vi "Main.vi"() -> ()   [LabVIEW 2019]
uses:
  Global.vi
  <vilib>/Utility/file.llb/Read Delimited Spreadsheet (DBL).vi
panel:
  out "Absorbancs Graph":cluster{dbl[], dbl[]}[](graph)=[{[210.47, 211.013, 211.556, 212.099, 212.642, 213.185, 213.728, 214.271, 214.814, 215.357, 215.9, 216.443, 216.986, 217.529, 218.072, 218.615, 219.158, 219.701, 220.244, 220.787, 221.33, 221.873, 222.416, 222.959, 223.502, 224.045, 224.588, 225.131, 225.674, 226.217, 226.76, 227.303, 227.846, 228.389, 228.932, 229.475, 230.018, 230.561, 231.104, 231.647, 232.19, 232.733, 233.276, 233.819, 234.362, 234.905, 235.448, 235.991, 236.534, 237.077, 237.62, 238.163, 238.706, 239.249, 239.792, 240.335, 240.878, 241.421, 241.964, 242.507, 243.05, 243.593, 244.136, 244.679, 245.222, 245.765, 246.308, 246.851, 247.394, 247.937, 248.48, 249.023, 249.566, 250.109, 250.652, 251.195, 251.738, 252.281, 252.824, 253.367, 253.91, 254.453, 254.996, 255.539, 256.082, 256.625, 257.168, 257.711, 258.254, 258.797, 259.34, 259.883], [0.859775678286318, 0.8194318156296146, 0.7895662441158913, 0.7653583418970374, 0.7134020372603199, 0.6674930001591154, 0.6169042198464642, 0.5666594591614739, 0.5127610913357338, 0.4760432747417854, 0.43179210618385533, 0.39546521483677954, 0.35704563080021307, 0.3204937163802063, 0.2943543872023645, 0.2644968000756883, 0.23727151168709026, 0.21506292164762564, 0.19582373256481655, 0.17509578429484746, 0.15778012766612576, 0.14182714481381176, 0.12762613288942176, 0.11359011007339652, 0.10311798710231297, 0.0919810390323458, 0.08407740857125809, 0.07520310011257239, 0.06894533118889845, 0.06156116409513224, 0.054721465538073055, 0.04951119044573565, 0.04379079748078188, 0.040522877073344524, 0.03583986731239025, 0.03120271181313547, 0.02776368982361145, 0.024890944782316078, 0.021970298789674186, 0.019046917639680402, 0.017650784209329966, 0.014430138184920574, 0.012660635378348474, 0.010678518980179588, 0.00996203492854495, 0.00865803175790969, 0.007123137178893124, 0.006459897966245347, 0.005454774486390257, 0.004673433507016052, 0.00317899640396703, 0.002978638971630067, 0.0032063812554244536, 0.0025374593715086283, 0.0010371917010740805, 0.0013682683081331706, 0.0012338025827769855, 0.00044231588608750066, 0.0006576235447054053, 0.0003592638366740966, 3.86590865093725e-05, -5.462381588621987e-05, -0.00043697341233217557, 0.00028768565388054973, -0.0005029989692543549, -0.0003836845555745434, -2.1769830005107654e-05, -8.158566931395356e-05, -0.0012657429248070888, -0.0009881653780830016, -0.0006206450872670022, -0.0008460195763415369, -0.0008440728182035687, -0.0008541442548795249, 0.0003212150192799558, -0.00016824964081266214, -0.0006849404823446592, 0.0004342318774892516, 0.00025692780195036777, 0.00010544427557851802, 0.00044687325757008026, -0.00017318641138520594, -4.097812470797019e-05, -8.4835930852626e-05, -0.00032452033611190395, -0.0006147450240710922, 0.00011997159689319109, -0.00015409533396294056, 0.0006683040427777585, 0.00014999181500151976, 0.0010128166761367956, 0.0012425823150642307]}, {[210.47, 211.013, 211.556, 212.099, 212.642, 213.185, 213.728, 214.271, 214.814, 215.357, 215.9, 216.443, 216.986, 217.529, 218.072, 218.615, 219.158, 219.701, 220.244, 220.787, 221.33, 221.873, 222.416, 222.959, 223.502, 224.045, 224.588, 225.131, 225.674, 226.217, 226.76, 227.303, 227.846, 228.389, 228.932, 229.475, 230.018, 230.561, 231.104, 231.647, 232.19, 232.733, 233.276, 233.819, 234.362, 234.905, 235.448, 235.991, 236.534, 237.077, 237.62, 238.163, 238.706, 239.249, 239.792, 240.335, 240.878, 241.421, 241.964, 242.507, 243.05, 243.593, 244.136, 244.679, 245.222, 245.765, 246.308, 246.851, 247.394, 247.937, 248.48, 249.023, 249.566, 250.109, 250.652, 251.195, 251.738, 252.281, 252.824, 253.367, 253.91, 254.453, 254.996, 255.539, 256.082, 256.625, 257.168, 257.711, 258.254, 258.797, 259.34, 259.883], [0.801341170479744, 0.7542734132237421, 0.6980568093186122, 0.65420605249337, 0.591680060881281, 0.5299625392926228, 0.47702592078260647, 0.4255234062398998, 0.3711647669162868, 0.3228829251218208, 0.2827599748503002, 0.2434409059716668, 0.2119311833930049, 0.1798378791449536, 0.15402672866461736, 0.13094215234558915, 0.10931855345881111, 0.09491646684250218, 0.07742521143320874, 0.06462685612767415, 0.05592972771866379, 0.04553833460727783, 0.03699743050859016, 0.031488515184952236, 0.025748999955385175, 0.020904706258801094, 0.018642890097352365, 0.013432623513669001, 0.010553223074843139, 0.009115474310373156, 0.008106302412446732, 0.00717074031072442, 0.005744777726777169, 0.004893684096016718, 0.0031711878437890757, 0.0015769760381964641, 0.0017569164268725172, 0.001484919073282149, 0.00034167784506089136, 0.00042709614687959363, -0.00019894237181035043, -0.0002881289314805198, -0.0009673652556734837, -0.0011091138604324736, 0.000146281936226407, -0.0005078123746470216, -0.0006453921276296619, -0.00040921704838469547, -0.00025853371894282023, -5.8841081421987657e-05, -0.0008455489737523095, -0.0003666006559215444, -0.0001741794938470015, -9.572694367300863e-05, -0.00013418443402012092, -0.0004342119920670712, -2.785591609676813e-05, -0.0005634379748792259, 0.0004540623443782983, -5.8901234707184336e-05, -0.00013105680029032452, -0.0003600499082511144, -0.0003055170322483515, 0.00045608059860526365, -0.00013473988615758312, 0.0007354698007963102, 0.00032433285193672265, 0.0007906108278793178, 7.605421447198432e-05, 8.534654960939622e-05, 0.0006625762183634851, -0.0005709729804337961, -0.0010150816524892026, 0.0001368035849654524, -0.000687954722901625, -0.00014905489719789847, 0.00011942950940802693, 0.000443837174362572, 0.00026005063494623573, -0.00020446941719183195, 0.000928426415228837, 0.000149226286241394, 2.9499413362117644e-05, -4.747285768441287e-05, 0.00033451056635025456, -0.00033948938772015297, -0.00025802686603175473, -0.0010796627525889724, 8.508559467040183e-05, 0.00019199329640829516, -2.422754560728671e-05, 0.00012878794244869374]}, {[210.47, 211.013, 211.556, 212.099, 212.642, 213.185, 213.728, 214.271, 214.814, 215.357, 215.9, 216.443, 216.986, 217.529, 218.072, 218.615, 219.158, 219.701, 220.244, 220.787, 221.33, 221.873, 222.416, 222.959, 223.502, 224.045, 224.588, 225.131, 225.674, 226.217, 226.76, 227.303, 227.846, 228.389, 228.932, 229.475, 230.018, 230.561, 231.104, 231.647, 232.19, 232.733, 233.276, 233.819, 234.362, 234.905, 235.448, 235.991, 236.534, 237.077, 237.62, 238.163, 238.706, 239.249, 239.792, 240.335, 240.878, 241.421, 241.964, 242.507, 243.05, 243.593, 244.136, 244.679, 245.222, 245.765, 246.308, 246.851, 247.394, 247.937, 248.48, 249.023, 249.566, 250.109, 250.652, 251.195, 251.738, 252.281, 252.824, 253.367, 253.91, 254.453, 254.996, 255.539, 256.082, 256.625, 257.168, 257.711, 258.254, 258.797, 259.34, 259.883], [0.8349250299196103, 0.7985659782220785, 0.7554294716845671, 0.7039073271955195, 0.6643155846589284, 0.6159979981150474, 0.5705818180332749, 0.5241666942013795, 0.4664351446159479, 0.4314871898047554, 0.3889092668584453, 0.35397500896861966, 0.32082659223672977, 0.29058708622423546, 0.26100520078520395, 0.23636505571931815, 0.212374355658777, 0.1941007847601965, 0.17582536275176977, 0.15957915032302233, 0.14560551256364115, 0.13224949336973374, 0.11922368957919263, 0.1097629242038428, 0.10189705539077057, 0.0928971760093605, 0.08538635126587726, 0.07812652408738596, 0.07171836378664848, 0.06508217851129808, 0.060563676829728776, 0.0558150422512567, 0.052404168918151785, 0.04734459073599655, 0.043400995888894185, 0.03996295459186795, 0.03540756730509166, 0.033186749038576574, 0.029867698307559296, 0.027606079350583596, 0.024793568873241023, 0.02179476713041542, 0.019525144001637858, 0.01779689632707871, 0.016386094716066633, 0.014686993002350365, 0.012953061761290088, 0.011800535044244484, 0.009986607793191861, 0.008508683009597853, 0.007255921855678818, 0.005920522311633751, 0.005428452139574033, 0.004341510976025073, 0.003272882804573607, 0.002792275615607423, 0.002627046818162858, 0.001956247104735409, 0.001975511612610885, 0.0005299670100274712, 0.0004937405679766166, 0.0010159557259308144, -0.00043008610603853525, 0.00022898969989317702, -0.0009699640550975969, 5.282040887574779e-05, -0.0010025972441931735, -0.0006509174041809049, -0.0017295119228779299, -0.0026943110513844987, -0.0017292772649578902, -0.0011740793412730113, -0.0020890149910946926, -0.0026277233640298464, -0.0007945791770674893, -0.0006339544985643902, -0.0012460337713899386, -0.0006416045454584116, -0.0004387120217184681, -0.0007055787813360359, -0.00044316594100983486, -0.0006635248767982091, -0.0009792362292916634, -0.00013667933511483932, 0.0006261275336703967, -0.0005395860806047259, 0.00012159334130024124, 0.0010251084460011217, 0.0018025827427642638, 0.001831767211735412, 0.0024732113092995472, 0.002767192854815498]}]
  out "A'- Graph":cluster{dbl[], dbl[]}[](graph)=[{[210.47, 211.013, 211.556, 212.099, 212.642, 213.185, 213.728, 214.271, 214.814, 215.357, 215.9, 216.443, 216.986, 217.529, 218.072, 218.615, 219.158, 219.701, 220.244, 220.787, 221.33, 221.873, 222.416, 222.959, 223.502, 224.045, 224.588, 225.131, 225.674, 226.217, 226.76, 227.303, 227.846, 228.389, 228.932, 229.475, 230.018, 230.561, 231.104, 231.647, 232.19, 232.733, 233.276, 233.819, 234.362, 234.905, 235.448, 235.991, 236.534, 237.077, 237.62, 238.163, 238.706, 239.249, 239.792, 240.335, 240.878, 241.421, 241.964, 242.507, 243.05, 243.593, 244.136, 244.679, 245.222, 245.765, 246.308, 246.851, 247.394, 247.937, 248.48, 249.023, 249.566, 250.109, 250.652, 251.195, 251.738, 252.281, 252.824, 253.367, 253.91, 254.453, 254.996, 255.539, 256.082, 256.625, 257.168, 257.711, 258.254, 258.797, 259.34, 259.883], [0.12793016694096082, 0.1327881561828641, 0.13898634561838696, 0.12591972077414348, 0.14132650024267335, 0.14734372113403094, 0.1485442487837778, 0.14751986962096558, 0.1377505703158608, 0.1454257108067617, 0.13827874574091015, 0.1380955602332684, 0.13280214091499964, 0.13096155295962345, 0.1242263335792905, 0.12003173950478929, 0.11520703411258498, 0.10969549971555984, 0.1069423396107689, 0.10205574991791058, 0.09580016806982122, 0.09167882996708734, 0.08624690930416284, 0.08168334522252357, 0.07892496597610259, 0.07423828091165904, 0.06873855259983945, 0.06612583621347973, 0.06228574814736767, 0.056930857187937944, 0.05331141850375127, 0.049396798883806, 0.04725985884383318, 0.042960378591267154, 0.040558634335614574, 0.038548841416862094, 0.03383136521287019, 0.031853948056984105, 0.02956088014857819, 0.027222379512650333, 0.02497238017948171, 0.02205386048567311, 0.02039542923280995, 0.01879516854143684, 0.016254370606103935, 0.015144480862862991, 0.013534765266055699, 0.012169541069378806, 0.01021984544175458, 0.008561791484343755, 0.008019447576661586, 0.006251714332178242, 0.0055858813703053, 0.004428072374523385, 0.0033942758849625923, 0.0031852781299558422, 0.0026522707441254765, 0.0024666851934537033, 0.001563969608097927, 0.0005833772835681486, 0.0006126350464351532, 0.0013427440658959052, -0.0001526640434080166, -0.00018534269449400133, -0.0008475009717322837, -0.0006159477395225684, -0.0012976525297084872, -0.0013704938482608704, -0.001798765017845805, -0.0027720616232884314, -0.0023331635827748016, -0.0006534404274150182, -0.0011629877379098984, -0.0027525829787817795, -0.00016639630496898027, -0.0004977867659968762, -0.0013551881915035838, -0.0010474447563982889, -0.000676610158729499, -0.0005184402556335553, -0.0012932934214892246, -0.000800229631418983, -0.001006272911124815, -9.314949136806912e-05, 0.0003192583376444662, -0.00022800478420321665, 0.00035851885260999834, 0.00201693730327079, 0.0017243828096380077, 0.001655229240884793, 0.002495498904283519, 0.002648662191671046]}]
  out "ENo3- Graph":cluster{dbl[], dbl[]}[](graph)=[{[210.47, 211.013, 211.556, 212.099, 212.642, 213.185, 213.728, 214.271, 214.814, 215.357, 215.9, 216.443, 216.986, 217.529, 218.072, 218.615, 219.158, 219.701, 220.244, 220.787, 221.33, 221.873, 222.416, 222.959, 223.502, 224.045, 224.588, 225.131, 225.674, 226.217, 226.76, 227.303, 227.846, 228.389, 228.932, 229.475, 230.018, 230.561, 231.104, 231.647, 232.19, 232.733, 233.276, 233.819, 234.362, 234.905, 235.448, 235.991, 236.534, 237.077, 237.62, 238.163, 238.706, 239.249, 239.792, 240.335, 240.878, 241.421, 241.964, 242.507, 243.05, 243.593, 244.136, 244.679, 245.222, 245.765, 246.308, 246.851, 247.394, 247.937, 248.48, 249.023, 249.566, 250.109, 250.652, 251.195, 251.738, 252.281, 252.824, 253.367, 253.91, 254.453, 254.996, 255.539, 256.082, 256.625, 257.168, 257.711, 258.254, 258.797, 259.34, 259.883], [2945.330127801271, 2980.855275880313, 3436.2790959666113, 3769.744784933901, 3866.894510497265, 4084.8736146849583, 4023.379959193408, 3942.792626230383, 3841.4870174255007, 4000.655053294645, 3828.2175896632853, 3817.29963026311, 3602.043449269673, 3441.6817617479314, 3385.4779019137154, 3191.9094774780338, 3027.900988481217, 2827.916240006436, 2758.161391723025, 2559.4402139484487, 2352.543562902859, 2211.319435258279, 2071.254044684568, 1872.4985984661555, 1757.9755053965123, 1610.3756628618062, 1481.2220799419745, 1391.9041799350034, 1312.4602246379604, 1178.0792525407564, 1046.9242425921682, 950.4885917176833, 853.0143961733057, 798.0735127864109, 729.9870960192372, 660.3096910237371, 580.0703495049484, 521.9091337484808, 481.03639003988167, 414.2641235694944, 396.4369339279932, 326.7555408020507, 301.8030154403679, 260.7798205817484, 218.2783416579434, 203.17512601786376, 172.00088731688328, 152.2553896286287, 126.72119927733758, 105.10817416921849, 88.68612370915851, 74.02308578565034, 74.9778366321423, 58.43746750873835, 25.92479027667191, 39.72329096416452, 28.016242550079305, 21.946810990329947, 4.837550849460239, 9.253260306661115, 3.6872160631477606, 6.564562628975335, -3.102759697380701, -3.4822870243873694, -8.257001809816265, -24.48707752878695, -7.530208161604536, -19.009160404506808, -29.78370140188913, -23.819749647347457, -28.252299308214194, -6.325350510303438, 3.4461920657718994, -21.976730977680553, 22.220061147224676, -0.46747996303027756, -17.84505210776972, -0.11357589657642167, -0.01733438945422087, 6.851118545455417, -10.561490174616834, -7.145991484163017, -1.5631996144296523, -0.8338814015497948, -14.628189953991297, -6.125489805889719, 8.399819289346626, 20.594630435447556, 12.956187847181663, -0.9477195505370489, 23.047848091745728, 24.73487218805406]}]
  out "[NO3] Linear fit":dbl=39.51302180661577 format="%#_3g"
  in  "Path Length":dbl=1.0 format="%#_13g"
  in  "[NO3-]":dbl=4.5e-05 caption="Known Nitrate Concentration"
  in  "S(TS)":dbl=33.66 caption="Sample Water Salinity" format="%#_13g"
  in  "S(KN)":dbl=33.85 caption="Calibration Salinity" format="%#_13g"
  in  "T(KN)":dbl=21.0 caption="Calibration Temp Zero Nitrate" format="%#_13g"
  in  "S(Norm)":dbl=35.0 caption="Calibration Salinity" format="%#_13g"
  in  "T(TS)":dbl=20.0 caption="Test Sample Sea Water Temp" format="%#_13g"
  in  "T(ZN)":dbl=19.3 caption="Calibration Temp Zero Nitrate" format="%#_13g"
  in  "S(ZN)":dbl=36.052 caption="Zero Nitrate Sea Water  Salinity" format="%#_13g"
  in  "btnCalcNitrate":bool caption="Calculate Nitrate"
  in  "DAC":T1(tab)
  in  "numTS":i32=6 caption="Column # (Zero Indexed)"
  in  "numKN":i32=3 caption="Column # (Zero Indexed)"
  in  "numZN":i32=4 caption="Column # (Zero Indexed)"
  in  "numDI":i32=2 caption="Column # (Zero Indexed)"
  in  "numDark":i32=1 caption="Column # (Zero Indexed)"
  out "ledTS":bool caption="Done"
  out "ledKN":bool caption="Done"
  out "ledZN":bool caption="Done"
  out "ledDI":bool caption="Done"
  out "ledDark":bool caption="Done"
  in  "Path":path=path "C:/Users/Omid/Desktop/SIO 179/Nitrate/SIO179NitrateCalc/Data/DataSampled(11-12).csv"
  in  "btnReadFromFile":bool caption="Read from CSV file"
  out "Intensity Signal Graph":cluster{dbl[], dbl[]}[](graph)
  out "Intensity Graph":cluster{dbl[], dbl[]}[](graph)=[{[210.47, 211.013, 211.556, 212.099, 212.642, 213.185, 213.728, 214.271, 214.814, 215.357, 215.9, 216.443, 216.986, 217.529, 218.072, 218.615, 219.158, 219.701, 220.244, 220.787, 221.33, 221.873, 222.416, 222.959, 223.502, 224.045, 224.588, 225.131, 225.674, 226.217, 226.76, 227.303, 227.846, 228.389, 228.932, 229.475, 230.018, 230.561, 231.104, 231.647, 232.19, 232.733, 233.276, 233.819, 234.362, 234.905, 235.448, 235.991, 236.534, 237.077, 237.62, 238.163, 238.706, 239.249, 239.792, 240.335, 240.878, 241.421, 241.964, 242.507, 243.05, 243.593, 244.136, 244.679, 245.222, 245.765, 246.308, 246.851, 247.394, 247.937, 248.48, 249.023, 249.566, 250.109, 250.652, 251.195, 251.738, 252.281, 252.824, 253.367, 253.91, 254.453, 254.996, 255.539, 256.082, 256.625, 257.168, 257.711, 258.254, 258.797, 259.34, 259.883], [2945.330127801271, 2980.855275880313, 3436.2790959666113, 3769.744784933901, 3866.894510497265, 4084.8736146849583, 4023.379959193408, 3942.792626230383, 3841.4870174255007, 4000.655053294645, 3828.2175896632853, 3817.29963026311, 3602.043449269673, 3441.6817617479314, 3385.4779019137154, 3191.9094774780338, 3027.900988481217, 2827.916240006436, 2758.161391723025, 2559.4402139484487, 2352.543562902859, 2211.319435258279, 2071.254044684568, 1872.4985984661555, 1757.9755053965123, 1610.3756628618062, 1481.2220799419745, 1391.9041799350034, 1312.4602246379604, 1178.0792525407564, 1046.9242425921682, 950.4885917176833, 853.0143961733057, 798.0735127864109, 729.9870960192372, 660.3096910237371, 580.0703495049484, 521.9091337484808, 481.03639003988167, 414.2641235694944, 396.4369339279932, 326.7555408020507, 301.8030154403679, 260.7798205817484, 218.2783416579434, 203.17512601786376, 172.00088731688328, 152.2553896286287, 126.72119927733758, 105.10817416921849, 88.68612370915851, 74.02308578565034, 74.9778366321423, 58.43746750873835, 25.92479027667191, 39.72329096416452, 28.016242550079305, 21.946810990329947, 4.837550849460239, 9.253260306661115, 3.6872160631477606, 6.564562628975335, -3.102759697380701, -3.4822870243873694, -8.257001809816265, -24.48707752878695, -7.530208161604536, -19.009160404506808, -29.78370140188913, -23.819749647347457, -28.252299308214194, -6.325350510303438, 3.4461920657718994, -21.976730977680553, 22.220061147224676, -0.46747996303027756, -17.84505210776972, -0.11357589657642167, -0.01733438945422087, 6.851118545455417, -10.561490174616834, -7.145991484163017, -1.5631996144296523, -0.8338814015497948, -14.628189953991297, -6.125489805889719, 8.399819289346626, 20.594630435447556, 12.956187847181663, -0.9477195505370489, 23.047848091745728, 24.73487218805406]}]
  out "ledSampledStatus":bool caption="Sampling is done!!"
  in  "Variable Selector":string(combo)="Dark Signal"
  in  "btnSampleFromSpectrometer":bool caption="Sample Signal From Spectrometer"
  out "ledSalinitySampledStatus":bool caption="Sampling is done!"
  in  "cmbSalinityVariableSelector":string(combo) caption="Variable Selector"
  in  "btnReadFromSalinitySensor":bool caption="Read from Salinity sensor"
  in  "baud rate":u32=9600 caption="Baud Rate"
  in  "Port Name":refnum<visa-resource-name>="COM1"
  in  "stop":bool
  # "Dark Signal"
  # "DI Water Signal"
  # "Zero Nitrate Signal"
  # "Known Nitrate Signal"
  # "Test Sample Signal"
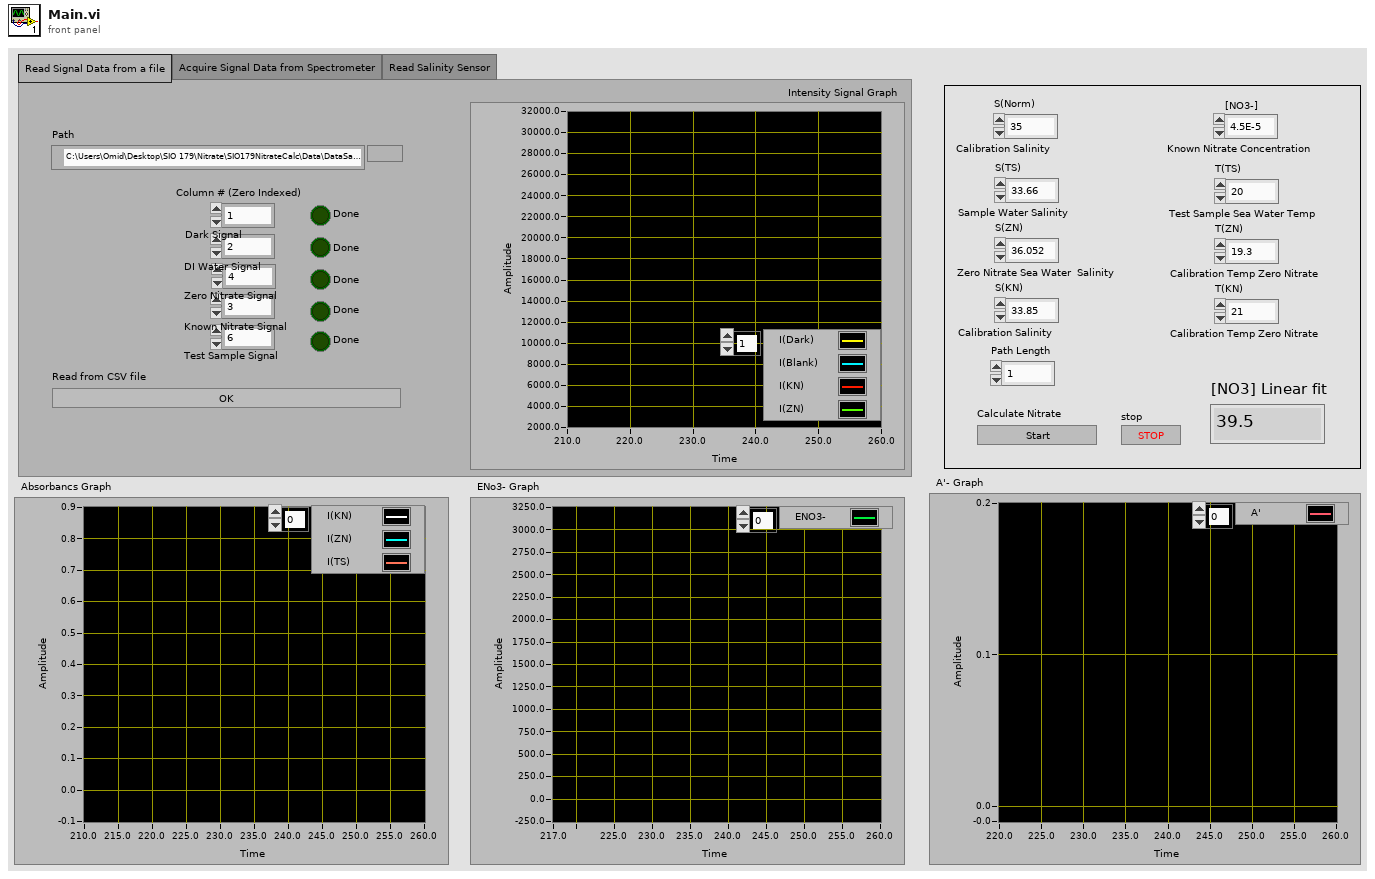
[diagram p1: front panel]
types:
  T1 = enum32{"Read Signal Data from a file", "Acquire Signal Data from Spectrometer", "Read Salinity Sensor"}
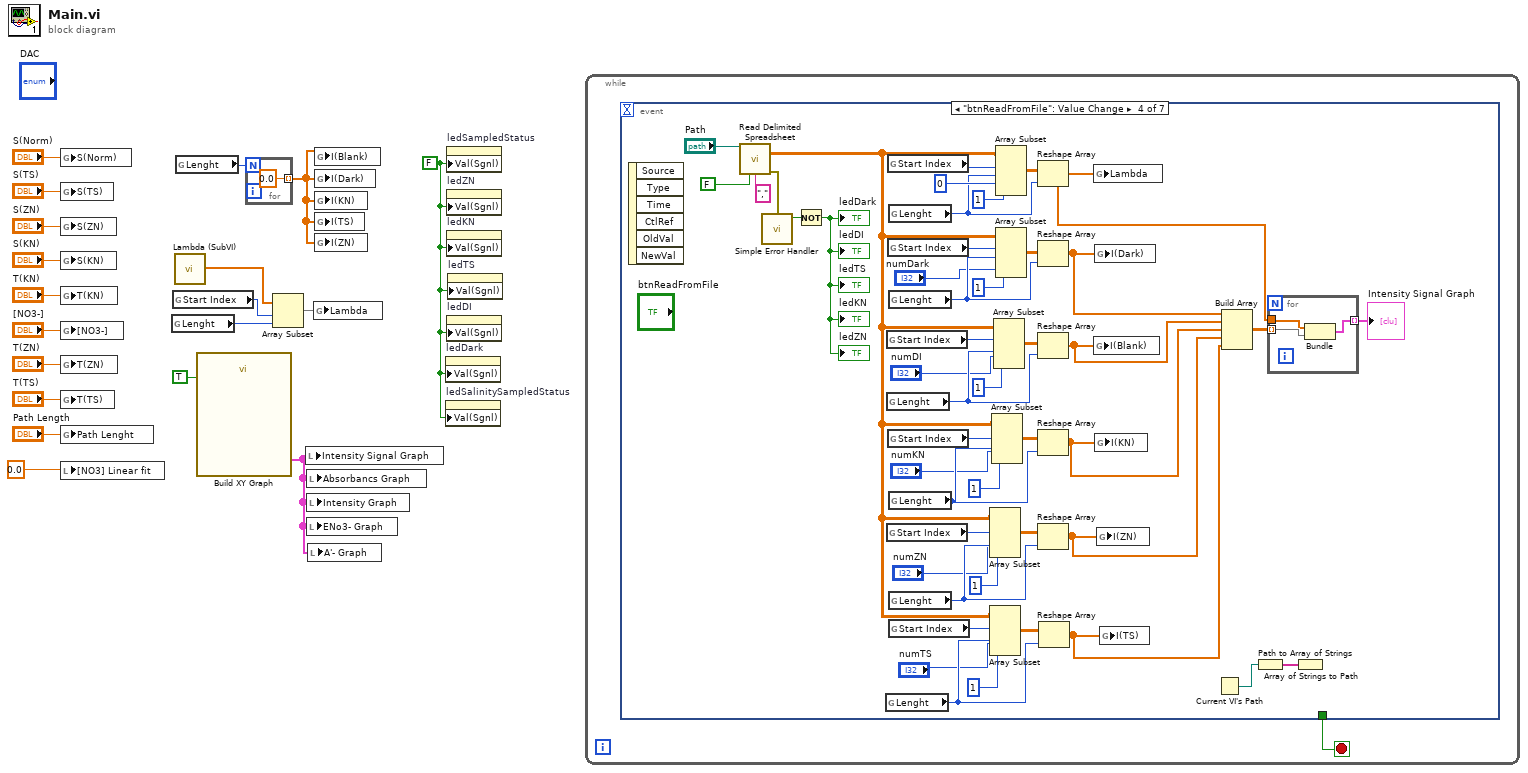
[diagram p0: block diagram]
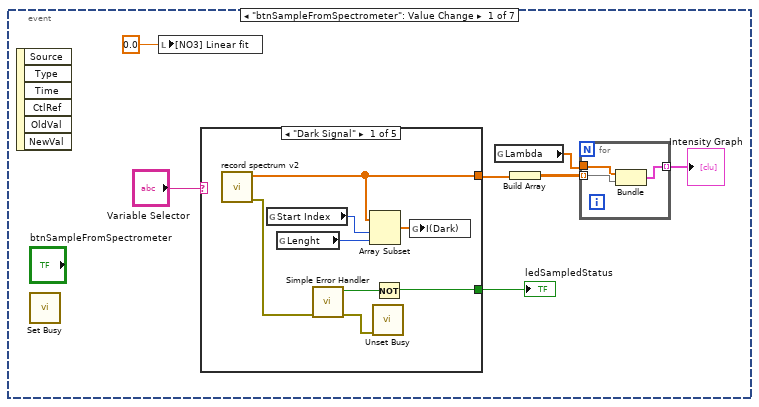
[diagram p2: hidden frame]
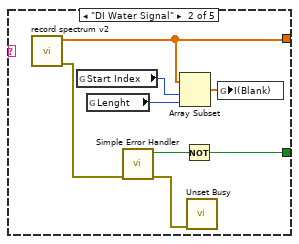
[diagram p3: hidden frame]
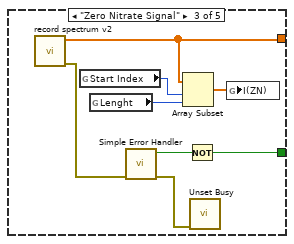
[diagram p4: hidden frame]
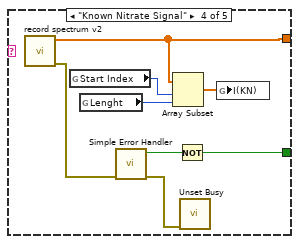
[diagram p5: hidden frame]
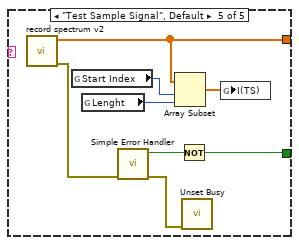
[diagram p6: hidden frame]
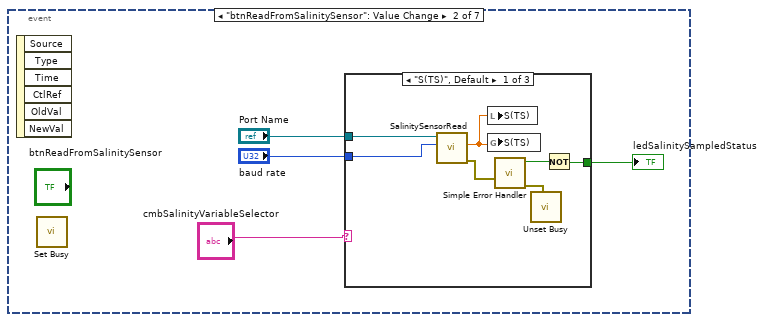
[diagram p7: hidden frame]
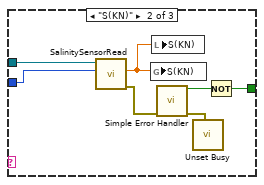
[diagram p8: hidden frame]
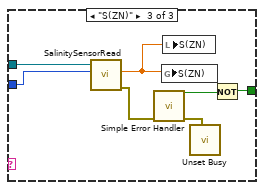
[diagram p9: hidden frame]
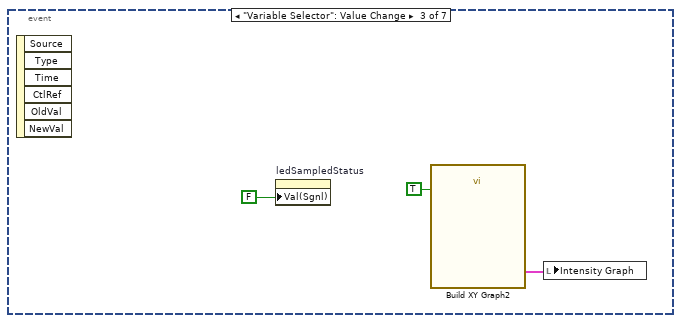
[diagram p10: hidden frame]
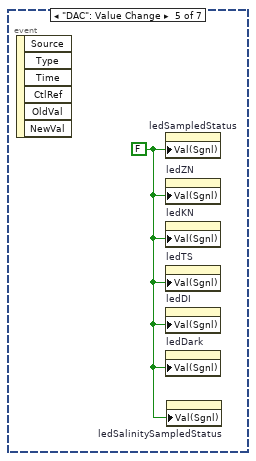
[diagram p11: hidden frame]
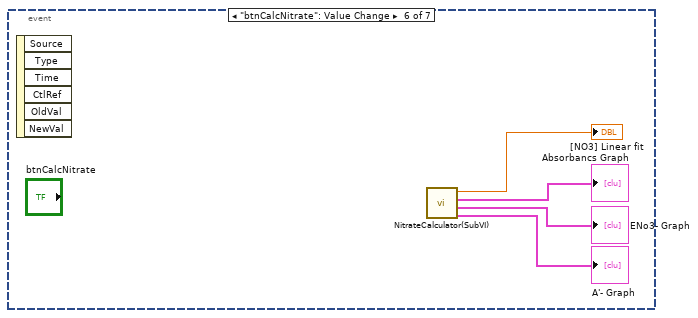
[diagram p12: hidden frame]
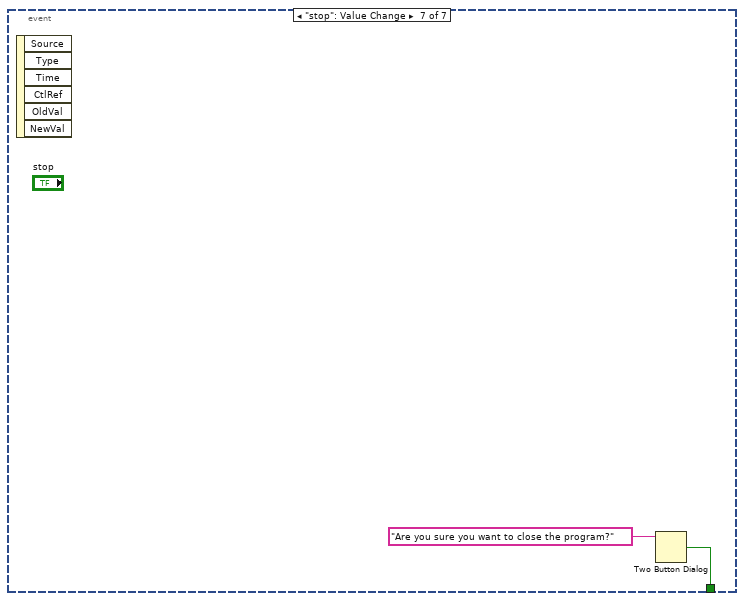
[diagram p13: hidden frame]
diagram:
  w10 = FALSE ("Value (Signaling)")
  n1 = global write "Global.vi" "S(Norm)"("S(Norm)") -> ()
  n2 = global write "Global.vi" "S(TS)"("S(TS)") -> ()
  n3 = global write "Global.vi" "S(ZN)"("S(ZN)") -> ()
  n4 = global write "Global.vi" "S(KN)"("S(KN)") -> ()
  n5 = global write "Global.vi" "T(KN)"("T(KN)") -> ()
  n6 = global write "Global.vi" "[NO3-]"("[NO3-]") -> ()
  n7 = global write "Global.vi" "T(ZN)"("T(ZN)") -> ()
  n8 = global write "Global.vi" "T(TS)"("T(TS)") -> ()
  n9 = global write "Global.vi" "Path Lenght"("Path Length") -> ()
  n10 = local write "[NO3] Linear fit"(0.0 ("[NO3] Linear fit")) -> ()
  n11 = global read "Global.vi" "Lenght"() -> (w16:i32)
  n12 = global read "Global.vi" "Start Index"() -> (w15:i32)
  n13 = call "Lambda (SubVI).vi"() -> ("Lambda"=w13:dbl[])  [unwired: 11 in]
  n14 = global read "Global.vi" "Lenght"() -> (w12:i32)
  n15 = call "Build XY Graph"("Reset"=TRUE) -> ("XY Graph"=w19:cluster{"Y":dbl[], "Y":dbl[]}[])  [unwired: 4 in, 6 out]
  n16 = for {
    N: w12 -> [_]
    tunnel: [0.0] -> w11 mode=indexing
  }
  n17 = Array Subset(array=w13, index=w15, length=w16) -> (w14:dbl[])
  n18 = local write "Intensity Signal Graph"(w19) -> ()
  n19 = local write "Absorbancs Graph"(w19) -> ()
  n20 = local write "Intensity Graph"(w19) -> ()
  n21 = local write "ENo3- Graph"(w19) -> ()
  n22 = local write "A'- Graph"(w19) -> ()
  n23 = global write "Global.vi" "Lambda"(w14) -> ()
  n24 = global write "Global.vi" "I(Blank)"(w11) -> ()
  n25 = global write "Global.vi" "I(Dark)"(w11) -> ()
  n26 = global write "Global.vi" "I(KN)"(w11) -> ()
  n27 = global write "Global.vi" "I(TS)"(w11) -> ()
  n28 = global write "Global.vi" "I(ZN)"(w11) -> ()
  n29 = property on="ledDark" class="Bool (strict)"("Val(Sgnl)"=w10) -> ()  [unwired: 2 in, 2 out]
  n30 = property on="ledSalinitySampledStatus" class="Bool (strict)"("Val(Sgnl)"=w10) -> ()  [unwired: 2 in, 2 out]
  n31 = property on="ledSampledStatus" class="Bool (strict)"("Val(Sgnl)"=w10) -> ()  [unwired: 2 in, 2 out]
  n32 = property on="ledZN" class="Bool (strict)"("Val(Sgnl)"=w10) -> ()  [unwired: 2 in, 2 out]
  n33 = property on="ledKN" class="Bool (strict)"("Val(Sgnl)"=w10) -> ()  [unwired: 2 in, 2 out]
  n34 = property on="ledDI" class="Bool (strict)"("Val(Sgnl)"=w10) -> ()  [unwired: 2 in, 2 out]
  n35 = property on="ledTS" class="Bool (strict)"("Val(Sgnl)"=w10) -> ()  [unwired: 2 in, 2 out]
  n36 = while {
    stop <- w21 stop-if-true
    n37 = event shown="[3] \"btnReadFromFile\": Value Change" {
      selector: _ -> [_ _ _ _ _ _ _]
      dyn-events: _ -> [_ _ _ _ _ _ _]
      timeout: _ -> [_ _ _ _ _ _ _]
      tunnel: [_ _ _ _ _ _ w156] -> w21
      event "btnSampleFromSpectrometer": Value Change {
        n38 = event-data() -> ()  [unwired: 1 in, 6 out]
        n39 = call <vilib>:"Set Busy.vi"() -> ()  [unwired: 10 in, 2 out]
        n40 = local write "[NO3] Linear fit"(0.0 ("[NO3] Linear fit")) -> ()
        n41 = case shown="\"Dark Signal\"" "Variable Selector" {
          tunnel: [w32 w40 w48 w56 w70] -> w27
          tunnel: [w33 w41 w49 w57 w64] -> w24
          frame "Dark Signal" {
            n42 = call "record spectrum v2.vi"() -> ("error out"=w36:errorcluster, "Array"=w33:dbl[])  [unwired: 9 in, 1 out]
            n43 = global read "Global.vi" "Start Index"() -> (w37:i32)
            n44 = global read "Global.vi" "Lenght"() -> (w38:i32)
            n45 = call <vilib>:"Simple Error Handler.vi"("error in (no error)"=w36) -> ("error?"=w34:bool, "error out"=w35:errorcluster)  [unwired: 4 in, 3 out]
            n46 = Array Subset(array=w33, index=w37, length=w38) -> (w39:dbl[])
            n47 = call <vilib>:"Unset Busy.vi"("error in (no error)"=w35) -> ()  [unwired: 10 in, 1 out]
            n48 = Not(x=w34) -> (.not. x?=w32:bool)
            n49 = global write "Global.vi" "I(Dark)"(w39) -> ()
          }
          frame "DI Water Signal" {
            n50 = call "record spectrum v2.vi"() -> ("error out"=w45:errorcluster, "Array"=w41:dbl[])  [unwired: 9 in, 1 out]
            n51 = global read "Global.vi" "Start Index"() -> (w44:i32)
            n52 = global read "Global.vi" "Lenght"() -> (w43:i32)
            n53 = call <vilib>:"Simple Error Handler.vi"("error in (no error)"=w45) -> ("error?"=w47:bool, "error out"=w46:errorcluster)  [unwired: 4 in, 3 out]
            n54 = Array Subset(array=w41, index=w44, length=w43) -> (w42:dbl[])
            n55 = Not(x=w47) -> (.not. x?=w40:bool)
            n56 = call <vilib>:"Unset Busy.vi"("error in (no error)"=w46) -> ()  [unwired: 10 in, 1 out]
            n57 = global write "Global.vi" "I(Blank)"(w42) -> ()
          }
          frame "Zero Nitrate Signal" {
            n58 = call "record spectrum v2.vi"() -> ("error out"=w53:errorcluster, "Array"=w49:dbl[])  [unwired: 9 in, 1 out]
            n59 = global read "Global.vi" "Start Index"() -> (w52:i32)
            n60 = global read "Global.vi" "Lenght"() -> (w51:i32)
            n61 = call <vilib>:"Simple Error Handler.vi"("error in (no error)"=w53) -> ("error?"=w55:bool, "error out"=w54:errorcluster)  [unwired: 4 in, 3 out]
            n62 = Array Subset(array=w49, index=w52, length=w51) -> (w50:dbl[])
            n63 = Not(x=w55) -> (.not. x?=w48:bool)
            n64 = call <vilib>:"Unset Busy.vi"("error in (no error)"=w54) -> ()  [unwired: 10 in, 1 out]
            n65 = global write "Global.vi" "I(ZN)"(w50) -> ()
          }
          frame "Known Nitrate Signal" {
            n66 = call "record spectrum v2.vi"() -> ("error out"=w61:errorcluster, "Array"=w57:dbl[])  [unwired: 9 in, 1 out]
            n67 = global read "Global.vi" "Start Index"() -> (w60:i32)
            n68 = global read "Global.vi" "Lenght"() -> (w59:i32)
            n69 = call <vilib>:"Simple Error Handler.vi"("error in (no error)"=w61) -> ("error?"=w63:bool, "error out"=w62:errorcluster)  [unwired: 4 in, 3 out]
            n70 = Array Subset(array=w57, index=w60, length=w59) -> (w58:dbl[])
            n71 = Not(x=w63) -> (.not. x?=w56:bool)
            n72 = call <vilib>:"Unset Busy.vi"("error in (no error)"=w62) -> ()  [unwired: 10 in, 1 out]
            n73 = global write "Global.vi" "I(KN)"(w58) -> ()
          }
          frame "Test Sample Signal", Default {
            n74 = call "record spectrum v2.vi"() -> ("error out"=w68:errorcluster, "Array"=w64:dbl[])  [unwired: 9 in, 1 out]
            n75 = global read "Global.vi" "Start Index"() -> (w67:i32)
            n76 = global read "Global.vi" "Lenght"() -> (w66:i32)
            n77 = call <vilib>:"Simple Error Handler.vi"("error in (no error)"=w68) -> ("error?"=w71:bool, "error out"=w69:errorcluster)  [unwired: 4 in, 3 out]
            n78 = Array Subset(array=w64, index=w67, length=w66) -> (w65:dbl[])
            n79 = Not(x=w71) -> (.not. x?=w70:bool)
            n80 = call <vilib>:"Unset Busy.vi"("error in (no error)"=w69) -> ()  [unwired: 10 in, 1 out]
            n81 = global write "Global.vi" "I(TS)"(w65) -> ()
          }
        }
        "ledSampledStatus" <- w27
        n82 = global read "Global.vi" "Lambda"() -> (w25:dbl[])
        n83 = Build Array(w24) -> (w26:dbl[][])
        n84 = for {
          tunnel: w26 -> [w31] mode=indexing
          tunnel: [w30] -> w23 mode=indexing
          tunnel: w25 -> [w29]
          n85 = Bundle("Lambda"=w29, w31) -> (w30:cluster{"Lambda":dbl[], dbl[]})  [unwired: 1 in]
        }
        "Intensity Graph" <- w23
      }
      event "btnReadFromSalinitySensor": Value Change {
        n86 = event-data() -> ()  [unwired: 1 in, 6 out]
        n87 = call <vilib>:"Set Busy.vi"() -> ()  [unwired: 10 in, 2 out]
        n88 = case shown="\"S(TS)\", Default" "cmbSalinityVariableSelector" {
          tunnel: "baud rate" -> [w82 w88 w95]
          tunnel: "Port Name" -> [w81 w89 w96]
          tunnel: [w77 w84 w91] -> w72
          frame "S(TS)", Default {
            n89 = call "SalinitySensorRead.vi"("VISA resource name"=w81, "baud rate"=w82) -> ("Salinity"=w76:dbl, "error out"=w78:errorcluster)  [unwired: 6 in, 1 out]
            n90 = local write "S(TS)"(w76) -> ()
            n91 = global write "Global.vi" "S(TS)"(w76) -> ()
            n92 = call <vilib>:"Simple Error Handler.vi"("error in (no error)"=w78) -> ("error?"=w79:bool, "error out"=w80:errorcluster)  [unwired: 4 in, 3 out]
            n93 = call <vilib>:"Unset Busy.vi"("error in (no error)"=w80) -> ()  [unwired: 10 in, 1 out]
            n94 = Not(x=w79) -> (.not. x?=w77:bool)
          }
          frame "S(KN)" {
            n95 = call "SalinitySensorRead.vi"("VISA resource name"=w89, "baud rate"=w88) -> ("Salinity"=w83:dbl, "error out"=w85:errorcluster)  [unwired: 6 in, 1 out]
            n96 = global write "Global.vi" "S(KN)"(w83) -> ()
            n97 = local write "S(KN)"(w83) -> ()
            n98 = call <vilib>:"Simple Error Handler.vi"("error in (no error)"=w85) -> ("error?"=w86:bool, "error out"=w87:errorcluster)  [unwired: 4 in, 3 out]
            n99 = call <vilib>:"Unset Busy.vi"("error in (no error)"=w87) -> ()  [unwired: 10 in, 1 out]
            n100 = Not(x=w86) -> (.not. x?=w84:bool)
          }
          frame "S(ZN)" {
            n101 = call "SalinitySensorRead.vi"("VISA resource name"=w96, "baud rate"=w95) -> ("Salinity"=w90:dbl, "error out"=w92:errorcluster)  [unwired: 6 in, 1 out]
            n102 = call <vilib>:"Simple Error Handler.vi"("error in (no error)"=w92) -> ("error?"=w94:bool, "error out"=w93:errorcluster)  [unwired: 4 in, 3 out]
            n103 = global write "Global.vi" "S(ZN)"(w90) -> ()
            n104 = local write "S(ZN)"(w90) -> ()
            n105 = call <vilib>:"Unset Busy.vi"("error in (no error)"=w93) -> ()  [unwired: 10 in, 1 out]
            n106 = Not(x=w94) -> (.not. x?=w91:bool)
          }
        }
        "ledSalinitySampledStatus" <- w72
      }
      event "Variable Selector": Value Change {
        n107 = event-data() -> ()  [unwired: 1 in, 6 out]
        n108 = property on="ledSampledStatus" class="Bool (strict)"("Val(Sgnl)"=FALSE ("ledSampledStatus")) -> ()  [unwired: 2 in, 2 out]
        n109 = call "Build XY Graph2"("Reset"=TRUE) -> ("XY Graph"=w97:cluster{"Y":dbl[], "Y":dbl[]}[])  [unwired: 4 in, 6 out]
        n110 = local write "Intensity Graph"(w97) -> ()
      }
      event "btnReadFromFile": Value Change {
        n111 = event-data() -> ()  [unwired: 1 in, 6 out]
        n112 = call-poly <vilib>:"Read Delimited Spreadsheet.vi"("file path (dialog if empty)"="Path", "transpose? (F)"=FALSE, "delimiter (\\t)"="," ("delimiter (\\t)")) -> ("all rows"=w139:dbl[][], "error out"=w103:errorcluster)  [unwired: 7 in, 4 out]
        n113 = call <vilib>:"Simple Error Handler.vi"("error in (no error)"=w103) -> ("error?"=w102:bool)  [unwired: 4 in, 4 out]
        n114 = Not(x=w102) -> (.not. x?=→"ledKN" →"ledDI" →"ledTS" →"ledZN" →"ledDark":bool)
        n115 = global read "Global.vi" "Lenght"() -> (w121:i32)
        n116 = global read "Global.vi" "Start Index"() -> (w126:i32)
        n117 = global read "Global.vi" "Lenght"() -> (w119:i32)
        n118 = global read "Global.vi" "Start Index"() -> (w124:i32)
        n119 = global read "Global.vi" "Start Index"() -> (w130:i32)
        n120 = global read "Global.vi" "Start Index"() -> (w128:i32)
        n121 = global read "Global.vi" "Start Index"() -> (w125:i32)
        n122 = global read "Global.vi" "Lenght"() -> (w129:i32)
        n123 = global read "Global.vi" "Lenght"() -> (w127:i32)
        n124 = global read "Global.vi" "Lenght"() -> (w122:i32)
        n125 = global read "Global.vi" "Lenght"() -> (w120:i32)
        n126 = global read "Global.vi" "Start Index"() -> (w123:i32)
        n127 = Array Subset(array=w139, index (row)=w124, length (row)=w120, index (col)="numZN", length (col)=1 ("length")) -> (w131:dbl[][])
        n128 = Array Subset(array=w139, index (row)=w123, length (row)=w121, index (col)="numTS", length (col)=1 ("length")) -> (w138:dbl[][])
        n129 = Array Subset(array=w139, index (row)=w125, length (row)=w122, index (col)="numKN", length (col)=1 ("length")) -> (w132:dbl[][])
        n130 = Array Subset(array=w139, index (row)=w126, length (row)=w119, index (col)="numDI", length (col)=1 ("length")) -> (w133:dbl[][])
        n131 = Array Subset(array=w139, index (row)=w130, length (row)=w129, index (col)=0 ("index"), length (col)=1 ("length")) -> (w135:dbl[][])
        n132 = Array Subset(array=w139, index (row)=w128, length (row)=w127, index (col)="numDark", length (col)=1 ("length")) -> (w134:dbl[][])
        n133 = Reshape Array(w135, w129) -> (w117:dbl[])
        n134 = Reshape Array(w134, w127) -> (w116:dbl[])
        n135 = Reshape Array(w133, w119) -> (w115:dbl[])
        n136 = Reshape Array(w132, w122) -> (w114:dbl[])
        n137 = Reshape Array(w131, w120) -> (w113:dbl[])
        n138 = Reshape Array(w138, w121) -> (w112:dbl[])
        n139 = global write "Global.vi" "Lambda"(w117) -> ()
        n140 = global write "Global.vi" "I(Blank)"(w115) -> ()
        n141 = global write "Global.vi" "I(Dark)"(w116) -> ()
        n142 = global write "Global.vi" "I(KN)"(w114) -> ()
        n143 = global write "Global.vi" "I(ZN)"(w113) -> ()
        n144 = global write "Global.vi" "I(TS)"(w112) -> ()
        n145 = Current VI's Path() -> (path=w105:path)
        n146 = Build Array(w116, w115, w114, w113, w112) -> (w118:dbl[][])
        n147 = Path to Array of Strings(0:w105) -> (2:w104:string[])  [unwired: 1 out]
        n148 = for {
          tunnel: w118 -> [w149] mode=indexing
          tunnel: [w148] -> w100 mode=indexing
          tunnel: w117 -> [w147]
          n149 = Bundle(w147, w149) -> (w148:cluster{dbl[], dbl[]})  [unwired: 1 in]
        }
        "Intensity Signal Graph" <- w100
        n150 = Array of Strings to Path(0:w104) -> ()  [unwired: 1 in, 1 out]
      }
      event "DAC": Value Change {
        w150 = FALSE ("Value (Signaling)")
        n151 = event-data() -> ()  [unwired: 1 in, 6 out]
        n152 = property on="ledSampledStatus" class="Bool (strict)"("Val(Sgnl)"=w150) -> ()  [unwired: 2 in, 2 out]
        n153 = property on="ledZN" class="Bool (strict)"("Val(Sgnl)"=w150) -> ()  [unwired: 2 in, 2 out]
        n154 = property on="ledKN" class="Bool (strict)"("Val(Sgnl)"=w150) -> ()  [unwired: 2 in, 2 out]
        n155 = property on="ledTS" class="Bool (strict)"("Val(Sgnl)"=w150) -> ()  [unwired: 2 in, 2 out]
        n156 = property on="ledDI" class="Bool (strict)"("Val(Sgnl)"=w150) -> ()  [unwired: 2 in, 2 out]
        n157 = property on="ledDark" class="Bool (strict)"("Val(Sgnl)"=w150) -> ()  [unwired: 2 in, 2 out]
        n158 = property on="ledSalinitySampledStatus" class="Bool (strict)"("Val(Sgnl)"=w150) -> ()  [unwired: 2 in, 2 out]
      }
      event "btnCalcNitrate": Value Change {
        n159 = event-data() -> ()  [unwired: 1 in, 6 out]
        n160 = call "NitrateCalculator(SubVI).vi"() -> ("A'- Graph"=→"A'- Graph":cluster{dbl[], dbl[]}[], "ENo3- Graph"=→"ENo3- Graph":cluster{dbl[], dbl[]}[], "Absorbancs Graph"=→"Absorbancs Graph":cluster{dbl[], dbl[]}[], "[NO3] Linear fit"=→"[NO3] Linear fit":dbl)  [unwired: 8 in]
      }
      event "stop": Value Change {
        n161 = event-data() -> ()  [unwired: 1 in, 6 out]
        n162 = Two Button Dialog(message="Are you sure you want to close the program?") -> (T button?=w156:bool)  [unwired: 2 in]
      }
    }
  }
